vi "solar_qtimer Set EnQType.vi"(6 "Suppress Errors? (T)":bool=TRUE, 7 "Target Name":string, 8 "error in (no error)":errorcluster, 9 "EnQ_Type (IgnoreIfExists)":enum8{"Normal", "Priority", "IgnoreIfExists"}(ring)=enum."IgnoreIfExists", 10 "QTimer Name":string, 11 "QTimer Refnum in":T1) -> (0 "error out":errorcluster, 3 "QTimer Refnum out":T1)   [LabVIEW 2018]
doc: "This sets the enqueue type of the QTimer by name.\nIgnore If Exists: Does not enqueue the command if it already exists in the queue\nNormal: Always enqueues a new message\nPriority: Enqueues the message on the front of the queue."
uses:
  solar_qtimer_ctl Refnum.ctl
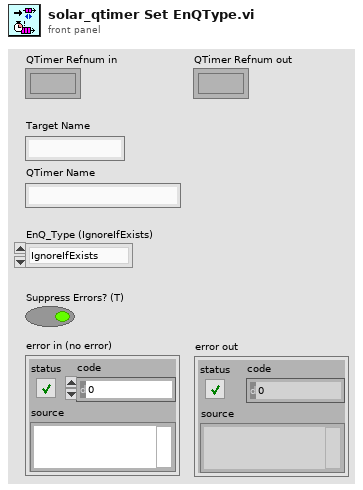
[diagram p1: front panel]
types:
  T1 = typedef "solar_qtimer_ctl Refnum.ctl" = refnum<k1>
  T2 = typedef "solar_qtimer_ctl SEQ.ctl" = cluster{"QTimers":T3[]}
  T3 = typedef "solar_qtimer_ctl QTimer.ctl" = cluster{"Settings":T4, "Queue":refnum<queue>, "QTimerQ":refnum<queue>, "VI Refnum":refnum<vi>}
  T4 = typedef "solar_qtimer_ctl QTimer Settings.ctl" = cluster{"QTimer":string, "Delay":i32, "Start":bool, "EnQ_Type":enum8{"Normal", "Priority", "IgnoreIfExists"}, "Messages":cluster{"MSG":string, "DATA":variant}[]}
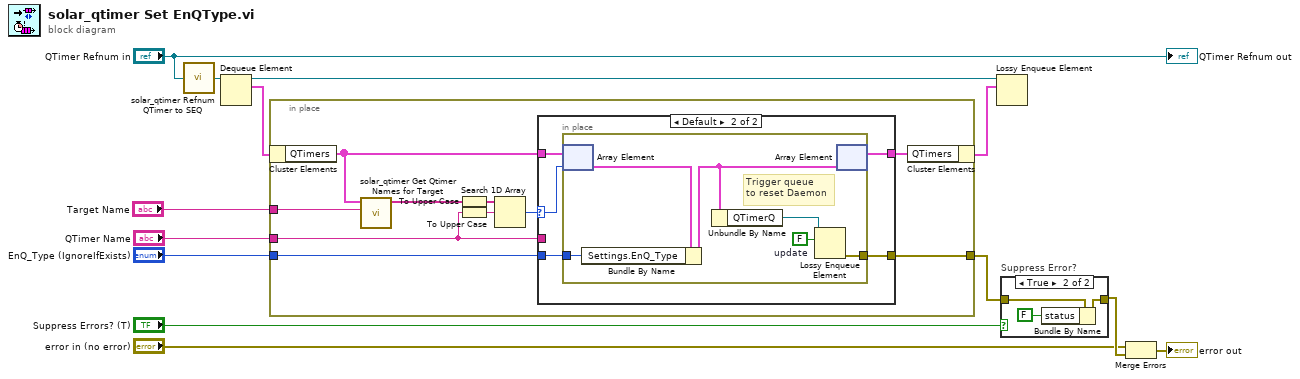
[diagram p0: block diagram]
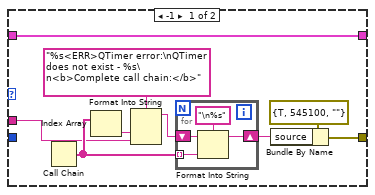
[diagram p2: hidden frame]
diagram:
  n1 = call "solar_qtimer Refnum QTimer to SEQ.vi"("QTimer Refnum"="QTimer Refnum in") -> ("QTimers SEQ"=w13:refnum<queue>)
  n2 = Dequeue Element(queue=w13) -> (queue out=w12:refnum<queue>, element=w11:T2)  [unwired: 2 in, 2 out]
  n3 = in-place {
    in-place-border: "QTimer Name" -> [w19]
    in-place-border: [w18] -> w7
    in-place-border: "EnQ_Type (IgnoreIfExists)" -> [w17]
    in-place-border: "Target Name" -> [w15]
    n4 = in-place-cluster #1(w11) -> ("QTimers"=w16:T3[])
    n5 = call "solar_qtimer Get Qtimer Names for Target.vi"("Target Name"=w15, "QTimers"=w16) -> ("Target's Qtimer Names"=w14:string[])  [unwired: 9 in]
    n6 = To Upper Case(1:w14) -> (0:w23:string[])
    n7 = To Upper Case(1:w19) -> (0:w22:string)
    n8 = Search 1D Array(1D array=w23, element=w22) -> (index of element=w21:i32)  [unwired: 1 in]
    n9 = case shown="Default" w21 {
      selector: w21 -> [_ w40]
      tunnel: w16 -> [w32 w41]
      tunnel: [w32 w39] -> w20
      tunnel: w19 -> [w25 _]
      tunnel: [w24 w37] -> w18
      tunnel: w17 -> [_ w38]
      frame -1 {
        n10 = Call Chain() -> (call chain=w28:string[])
        n11 = Index Array(array=w28) -> (element=w30:string)  [unwired: 1 in]
        n12 = Format Into String(format string="%s<ERR>QTimer error:\nQTimer does not exist - %s\n<b>Complete call chain:</b>", w30, w25) -> (resulting string=w29:string)  [unwired: 2 in, 1 out]
        n13 = for {
          tunnel: w28 -> [w36] mode=indexing
          shift-right: [w35] -> w27
          shift-left: w29 -> [w34]
          n14 = Format Into String(format string="\n%s", initial string=w34, w36) -> (resulting string=w35:string)  [unwired: 1 in, 1 out]
        }
        n15 = Bundle By Name(cluster=errorcluster {"status"=TRUE, "code"=545100, "source"=""} ("error in (no error)"), "source"=w27) -> (w24:errorcluster)
      }
      frame Default {
        n16 = in-place {
          in-place-border: w38 -> [w46]
          in-place-border: [w42] -> w37
          w43 = FALSE  # update
          # "Trigger queue\nto reset Daemon"
          n17 = in-place-array #2(w41, w40) -> (w47:T3)
          n18 = Bundle By Name(cluster=w47, "Settings.EnQ_Type"=w46) -> (w45:T3)
          n19 = Unbundle By Name(w45) -> ("QTimerQ"=w44:refnum<queue>)
          n20 = Lossy Enqueue Element(queue=w44, element=w43) -> (error out=w42:errorcluster)  [unwired: 1 in, 3 out]
          n21 = in-place-array #2(w45) -> (w39:T3[])  [unwired: 1 out]
        }
      }
    }
    n22 = in-place-cluster #1("QTimers"=w20) -> (w10:T2)
  }
  n23 = Lossy Enqueue Element(queue=w12, element=w10) -> ()  [unwired: 1 in, 4 out]
  n24 = case "Suppress Error?" shown="True" "Suppress Errors? (T)" {
    tunnel: w7 -> [w48 w51]
    tunnel: [w48 w50] -> w8
    frame False {
    }
    frame True {
      n25 = Bundle By Name(cluster=w51, "status"=FALSE) -> (w50:errorcluster)
    }
  }
  n26 = Merge Errors("error in (no error)", w8) -> (→"error out":errorcluster)
  "QTimer Refnum out" <- "QTimer Refnum in"
